vi "Get Event Structure Num.vi"(8 "error in (no error)":errorcluster, 11 "CSM-Helper in":refnum<class "CSM-Helper.lvclass">) -> (0 "error out":errorcluster, 2 "EvtStruNum":i32, 3 "CSM-Helper out":refnum<class "CSM-Helper.lvclass">)   [LabVIEW 2017, in "CSM-Helper.lvclass"]
doc: "### Get Event Structure Num.vi\n\n-- <b>Controls</b> --\n- <b>CSM-Helper in</b>: CSMHelper input\n\n-- <b>Indicators</b> --\n- <b>EvtStrutNum</b>:\n- <b>CSM-Helper out</b>: CSMHelper output"
uses:
  CSM-Helper.lvclass
  CSM-Helper.lvclass/CSM-Helper.ctl
  Properties/Read Case Structure Ref.vi
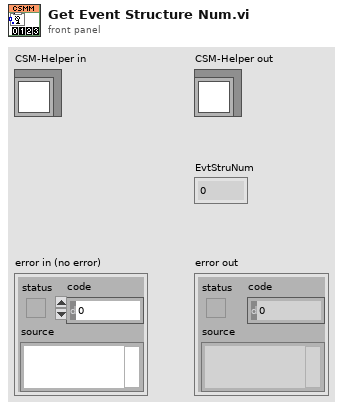
[diagram p1: front panel]
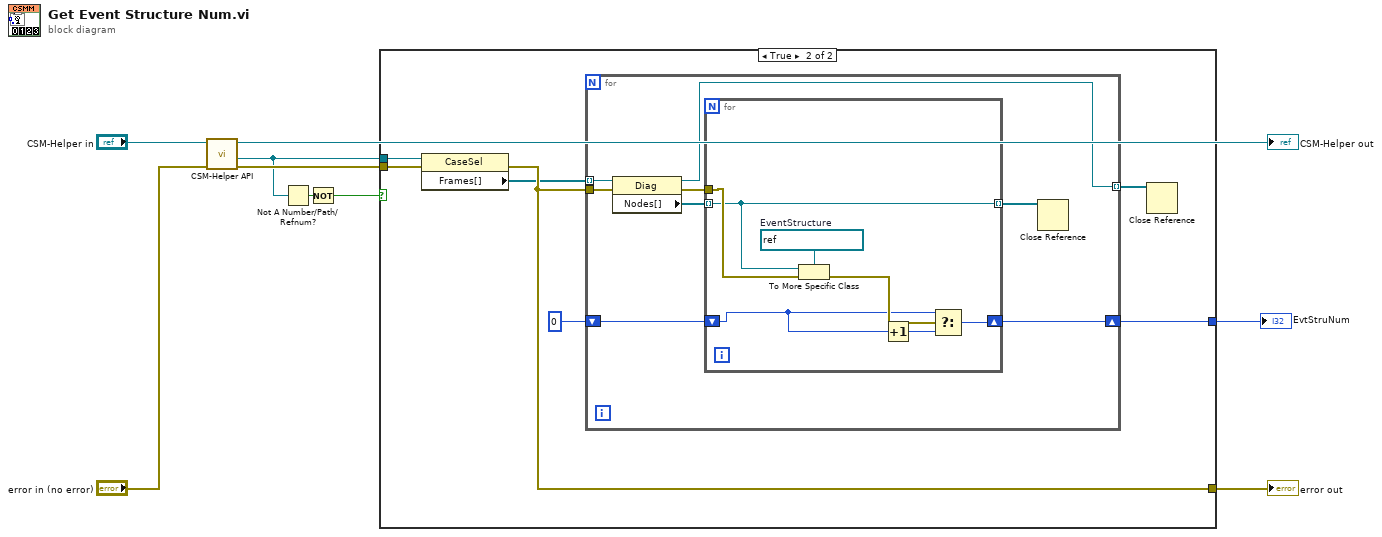
[diagram p0: block diagram]
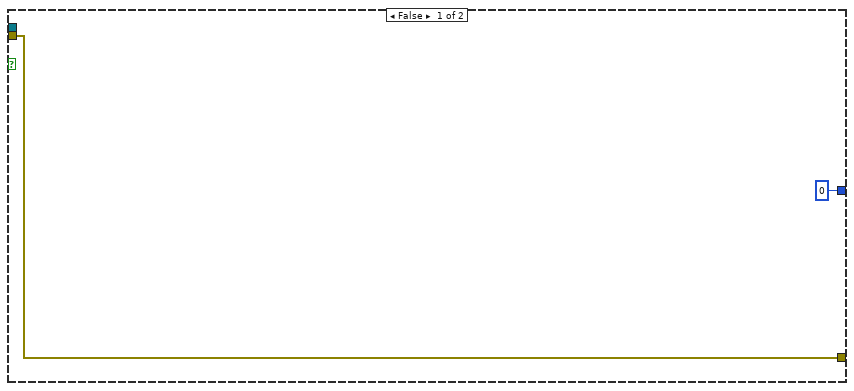
[diagram p2: hidden frame]
diagram:
  n1 = call-poly "CSM-Helper API.vi"("error in (no error)"="error in (no error)", "CSM-Helper in"="CSM-Helper in") -> ("error out"=w6:errorcluster, "Case Structure"=w3:refnum<vi>, "CSM-Helper out"=→"CSM-Helper out":refnum<class "CSM-Helper.lvclass">)  [unwired: 7 in]
  n2 = Not A Number/Path/Refnum?(number/path/refnum=w3) -> (NaN/Path/Refnum?=w2:bool)
  n3 = Not(x=w2) -> (.not. x?=w1:bool)
  n4 = case shown="True" w1 {
    tunnel: w6 -> [w11 w18]
    tunnel: [0 w16] -> w5
    tunnel: [w11 w15] -> w4
    tunnel: w3 -> [_ w12]
    frame False {
    }
    frame True {
      n5 = property class="CaseSel"(reference=w12, error in=w18) -> (error out=w15:errorcluster, "Frames[]"=w14:refnum<vi>[])  [unwired: 1 out]
      n6 = for {
        tunnel: w14 -> [w26] mode=indexing
        shift-right: [w24] -> w16
        shift-left: 0 -> [w25]
        tunnel: w15 -> [w22]
        tunnel: [w19] -> w13 mode=indexing
        n7 = property class="Diag"(reference=w26, error in=w22) -> (reference out=w19:refnum<vi>, error out=w21:errorcluster, "Nodes[]"=w23:refnum<vi>[])
        n8 = for {
          tunnel: w23 -> [w27] mode=indexing
          shift-right: [w32] -> w24
          shift-left: w25 -> [w30]
          tunnel: w21 -> [w28]
          tunnel: [w27] -> w20 mode=indexing
          w33 = refnum<vi> refnum  # EventStructure
          n9 = To More Specific Class(target class=w33, reference=w27, error in=w28) -> (error out=w31:errorcluster)  [unwired: 1 out]
          n10 = Increment(x=w30) -> (x+1=w29:i32)
          n11 = Select(t=w30, s=w31, f=w29) -> (s? t:f=w32:i32)
        }
        n12 = Close Reference(reference=w20) -> ()  [unwired: 1 in, 1 out]
      }
      n13 = Close Reference(reference=w13) -> ()  [unwired: 1 in, 1 out]
    }
  }
  "error out" <- w4
  "EvtStruNum" <- w5
